vi "Kepco cfg output mode.vi"(8 "error in (no error)":errorcluster {"code" format="%.0x"}, 9 "Simulation":T1, 10 "Channel parsed command info":T2, 11 "input cluster":refnum<class "KepcoBOP.lvclass">) -> (0 "error out":errorcluster, 2 "new commands":string, 3 "output cluster":refnum<class "KepcoBOP.lvclass">)   [LabVIEW 2020, in "KepcoBOP.lvclass"]
uses:
  KepcoBOP.lvclass
  channel parsed cmd cluster.ctl
  OnOffTypeDef.ctl
  KepcoBOP.lvclass/KepcoBOP.ctl
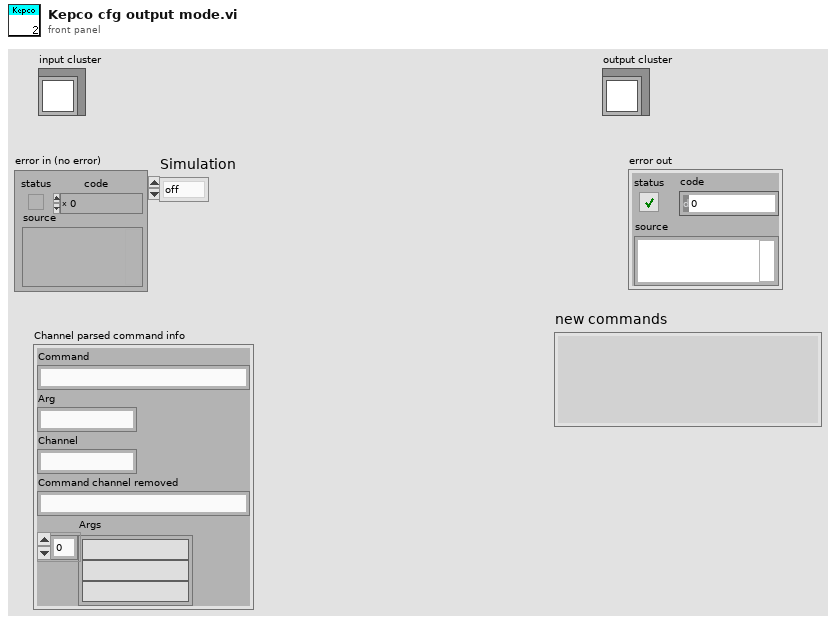
[diagram p1: front panel]
types:
  T1 = typedef "OnOffTypeDef.ctl" = enum16{"off", "on"}
  T2 = typedef "channel parsed cmd cluster.ctl" = cluster{"Command":string, "Arg":string, "Channel":string, "Command channel removed":string, "Args":string[]}
  T3 = enum16{"Fixed", "List", "Transient", "External", "Gain", "Protect", "Additive"}
  T4 = enum16{"Fixed", "List", "Transient", "External", "Gain", "Protect"}
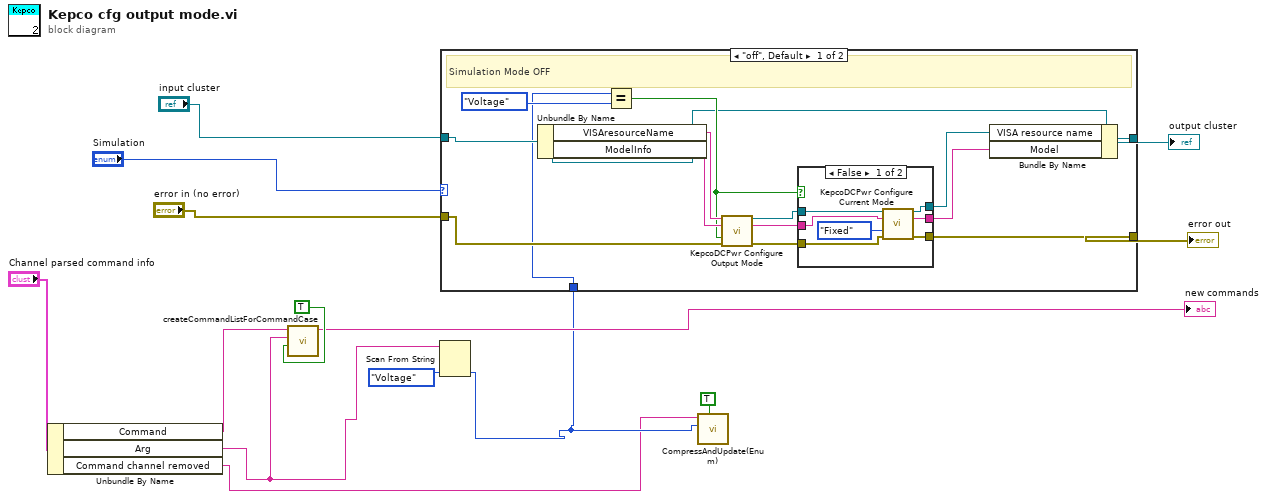
[diagram p0: block diagram]
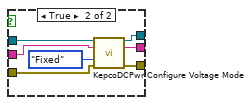
[diagram p2: hidden frame]
diagram:
  n1 = Unbundle By Name("Channel parsed command info") -> ("Command"=w2:string, "Arg"=w4:string, "Command channel removed"=w1:string)
  n2 = call "createCommandListForCommandCase.vi"("immediate Check (only once)"=TRUE, "setvalue"=w4, "command"=w2) -> ("new commands"=→"new commands":string)  [unwired: 8 in]
  n3 = Scan From String(input string=w4, default 1=enum16{"Voltage", "Current"}."Voltage") -> (output 1=w3:enum16{"Voltage", "Current"})  [unwired: 3 in, 3 out]
  n4 = case shown="\"off\", Default" "Simulation" {
    tunnel: [w16 w43] -> w9
    tunnel: w3 -> [w17 _]
    tunnel: "input cluster" -> [w18 w44]
    tunnel: "error in (no error)" -> [w19 w43]
    tunnel: [w15 w44] -> w10
    frame "off", Default {
      # "Simulation Mode OFF"
      n5 = Unbundle By Name(w18) -> ("VISAresourceName"=w28:string, "ModelInfo"=w27:string)
      n6 = Equal?(x=w17, y=enum16{"Voltage", "Current"}."Voltage") -> (x = y?=w26:bool)
      n7 = call "KepcoDCPwr Configure Output Mode.vi"("VISA Session"=w28, "Model In"=w27, "Mode In (Volt)"=w26, "error in (no error)"=w19) -> ("VISA Session Out"=w25:refnum<visa-resource-name>, "Model Out"=w21:string, "error out"=w24:errorcluster)  [unwired: 9 in]
      n8 = case shown="False" w26 {
        tunnel: w25 -> [w35 w42]
        tunnel: w24 -> [w33 w41]
        tunnel: [w32 w40] -> w16
        tunnel: [w34 w39] -> w23
        tunnel: [w29 w38] -> w22
        tunnel: w21 -> [w31 w37]
        frame False {
          n9 = call "KepcoDCPwr Configure Current Mode.vi"("VISA Session"=w35, "Model In"=w31, "Mode (Fixed)"=T3."Fixed", "error in (no error)"=w33) -> ("VISA Session Out"=w34:refnum<visa-resource-name>, "Model Out"=w29:string, "error out"=w32:errorcluster)  [unwired: 8 in, 1 out]
        }
        frame True {
          n10 = call "KepcoDCPwr Configure Voltage Mode.vi"("VISA Session"=w42, "Model In"=w37, "Mode (Fixed)"=T4."Fixed", "error in (no error)"=w41) -> ("VISA Session Out"=w39:refnum<visa-resource-name>, "Model Out"=w38:string, "error out"=w40:errorcluster)  [unwired: 8 in, 1 out]
        }
      }
      n11 = Bundle By Name(cluster=w18, "VISA resource name"=w23, "Model"=w22) -> (w15:refnum<class "KepcoBOP.lvclass">)
    }
    frame "on" {
      # "Simulation Mode ON"
    }
  }
  "output cluster" <- w10
  "error out" <- w9
  n12 = call "CompressAndUpdate(Enum).vi"("force CVT update (false)"=TRUE ("force CVT update"), "enum variant"=w3, "command or variable name"=w1) -> ()  [unwired: 8 in, 1 out]
